vi "Log Data Text.vi"(8 "Headers":string[](array[string])=["B (nT)", "Bx (nT)", "By (nT)", "Bz (nT)", "P (bar)", "T (C)", "ax (g)", "ay (g)", "az (g)", "gx (deg/s)", "gy (deg/s)", "gz (deg/s)"], 9 "format (%.3f)":string, 10 "Array":dbl[][](array[numeric]), 11 "Log to file":path) -> ()   [LabVIEW 2022 SP3]
uses:
  <vilib>/Utility/file.llb/Write Delimited Spreadsheet (DBL).vi
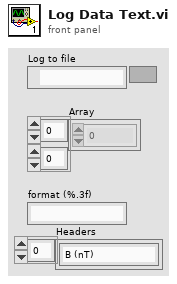
[diagram p1: front panel]
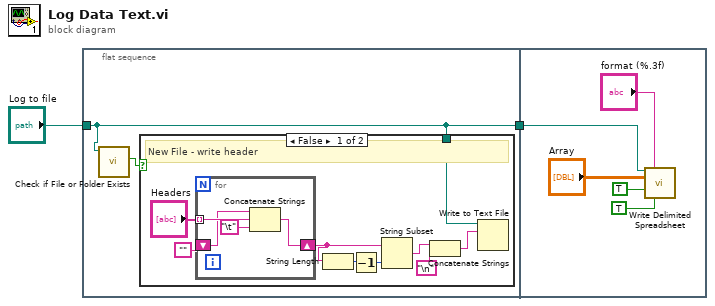
[diagram p0: block diagram]
diagram:
  n1 = flat-sequence {
    tunnel: "Log to file" -> [w3]
    tunnel: [w3] -> w1
    tunnel: w1 -> [w18]
    frame #0 {
      n2 = call <vilib>:"Check if File or Folder Exists.vi"("path"=w3) -> ("file or folder exists?"=w4:bool)  [unwired: 8 in, 2 out]
      n3 = case shown="False" w4 {
        tunnel: w3 -> [w5 _]
        frame False {
          # "New File - write header"
          n4 = for {
            tunnel: "Headers" -> [w17] mode=indexing
            shift-right: [w15] -> w11
            shift-left: "" -> [w14]
            n5 = Concatenate Strings(w14, w17, "\t") -> (w15:string)
          }
          n6 = String Length(string=w11) -> (length=w10:i32)
          n7 = Decrement(x=w10) -> (x-1=w9:i32)
          n8 = String Subset(string=w11, length (rest)=w9) -> (substring=w7:string)  [unwired: 1 in]
          n9 = Concatenate Strings(w7, "\n") -> (w6:string)
          n10 = Write to Text File(file (use dialog)=w5, text=w6) -> ()  [unwired: 2 in, 3 out]
        }
        frame True {
        }
      }
    }
    frame #1 {
      n11 = call-poly <vilib>:"Write Delimited Spreadsheet.vi"("file path (dialog if empty)"=w18, "format (%.3f)"="format (%.3f)", "2D data"="Array", "append to file? (new file:F)"=TRUE ("append to file? (F)"), "transpose? (no:F)"=TRUE ("transpose? (F)")) -> ()  [unwired: 9 in, 2 out]
    }
  }
